vi "ScanPanel.vi"(8 "error in (no error)":errorcluster caption="entrée d'erreur (pas d'erreur)", 11 "BaseDevice.lvclass":refnum<class "BaseDevice.lvclass">) -> (0 "error out":errorcluster caption="sortie d'erreur", 3 "BaseDevice.lvclass Out":refnum<class "BaseDevice.lvclass">)   [LabVIEW 2019, in "BaseDevice.lvclass"]
uses:
  BaseDevice.lvclass
  ScanPos.ctl
panel:
  in  "AllerRetour":bool
  in  "UpdateScanTime":bool
  in  "MainProgQ":refnum<queue>
  in  "MainProgQEvent":refnum<user-event>
  in  "Reinit":bool caption="Reinit. à la fin"
  in  "Bidir":bool
  out "Positions":dbl[](array[numeric])
  in  "Modèle":u16(ring) caption="Modèle de Balayage"
  in  "CréerMod":bool
  in  "Debut":dbl caption="Début"
  in  "Fin":dbl
  in  "Increment":dbl=inf
  in  "ModRap":bool caption="Modèle Rapide"
  in  "Stop":bool
  out "Init Program":bool
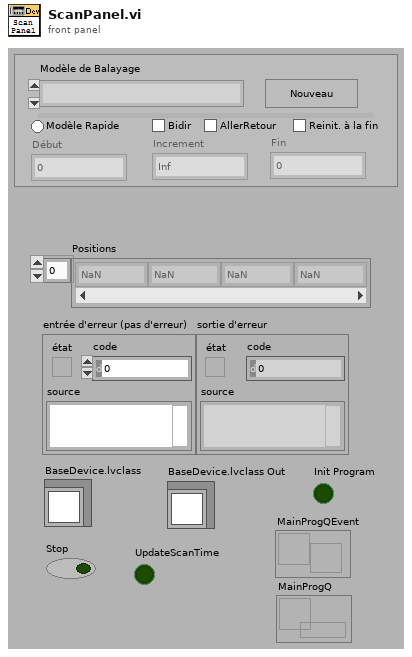
[diagram p1: front panel]
types:
  T1 = typedef "ScanPos.ctl" = cluster{"Debut":dbl, "Increment":dbl, "Fin":dbl, "Positions":dbl[], "Bidir":bool, "ModelRap":bool}
  T2 = enum16{"Enable", "Disable", "DisAndGrayed", "ReinitToDefVal"}
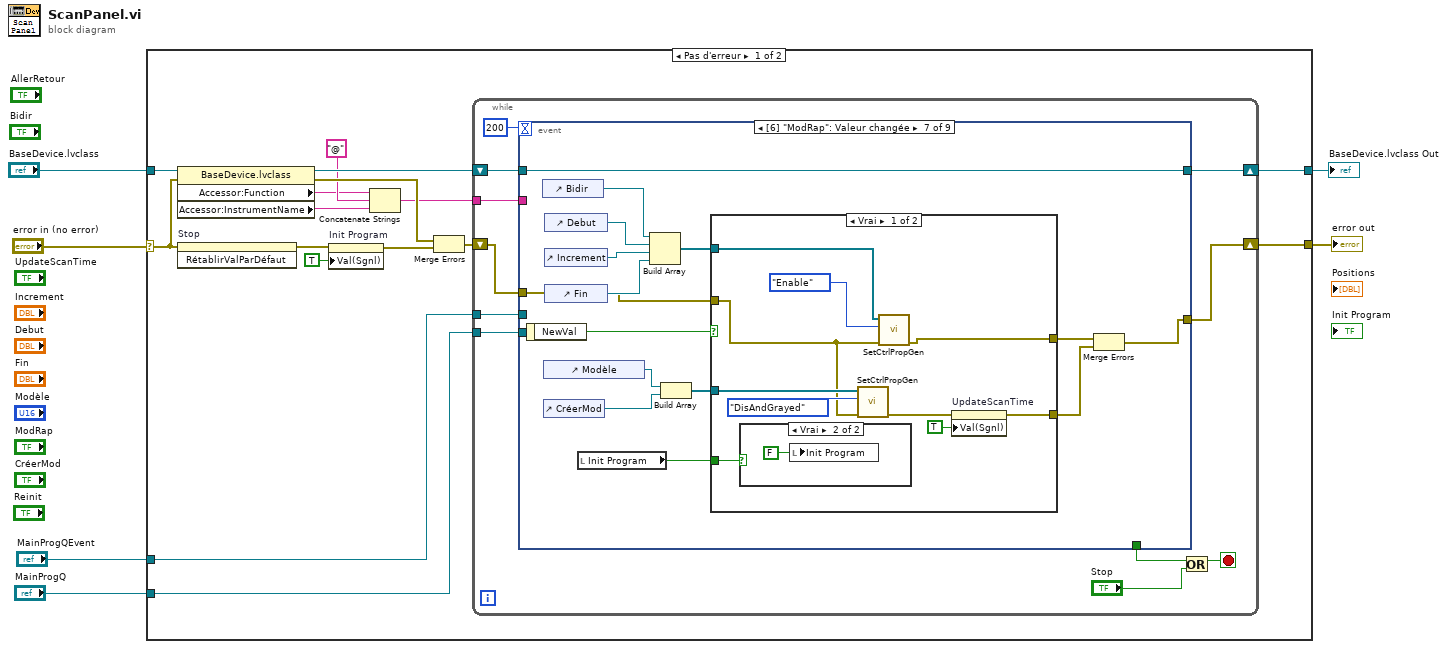
[diagram p0: block diagram]
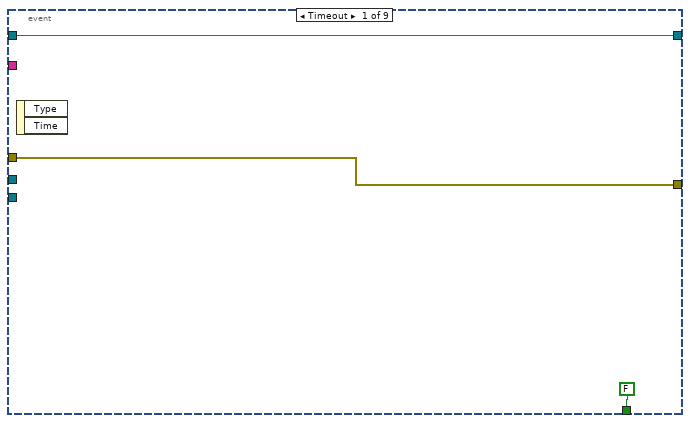
[diagram p2: hidden frame]
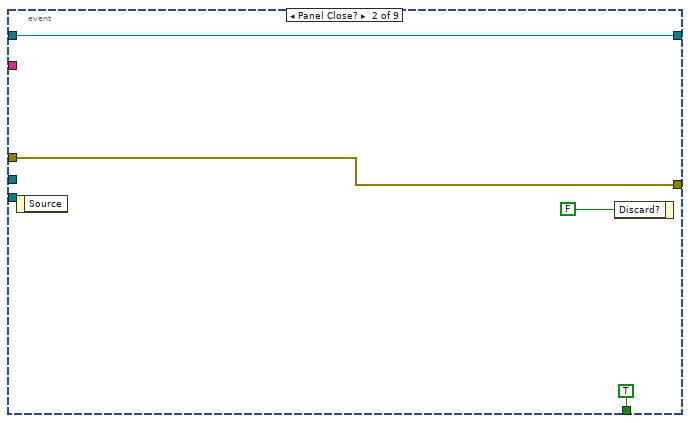
[diagram p3: hidden frame]
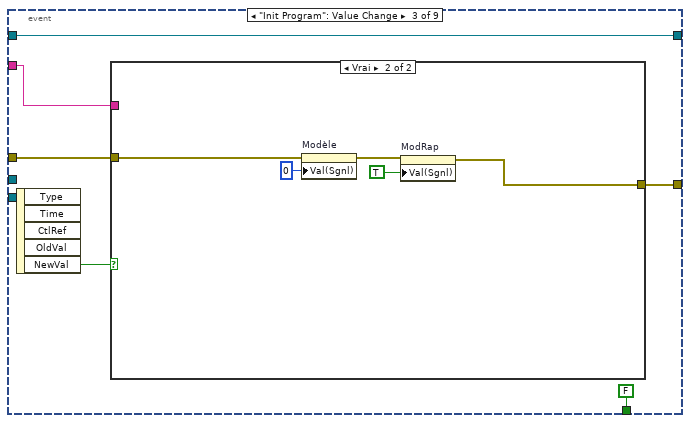
[diagram p4: hidden frame]
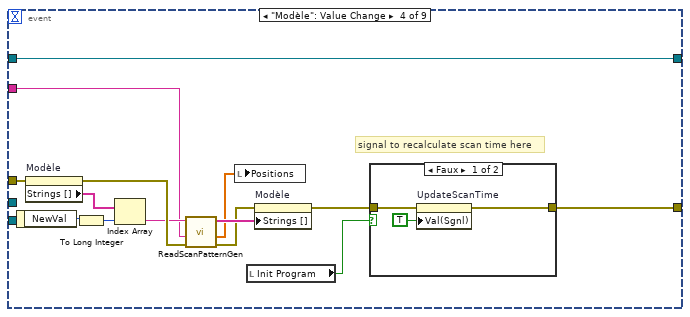
[diagram p6: hidden frame]
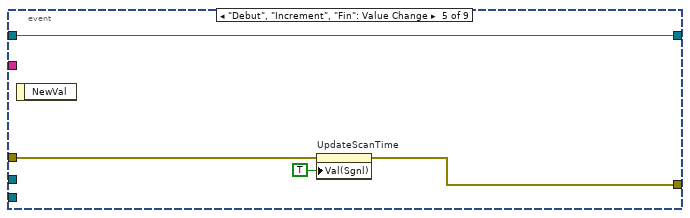
[diagram p8: hidden frame]
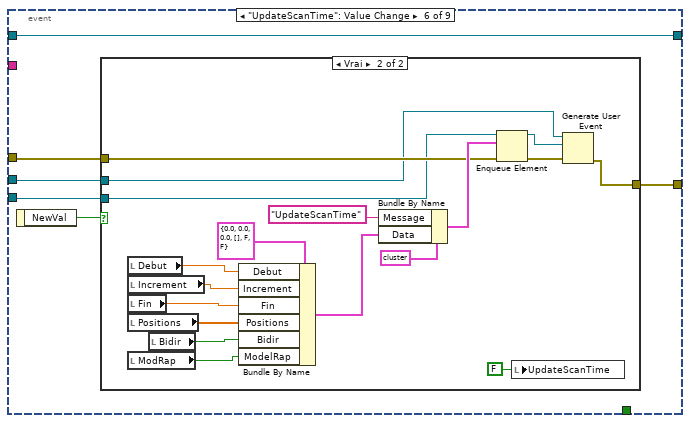
[diagram p9: hidden frame]
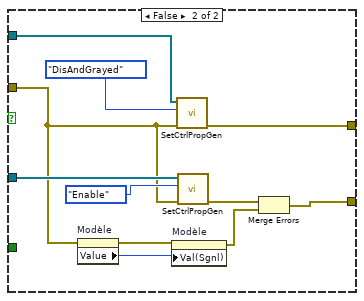
[diagram p12: hidden frame]
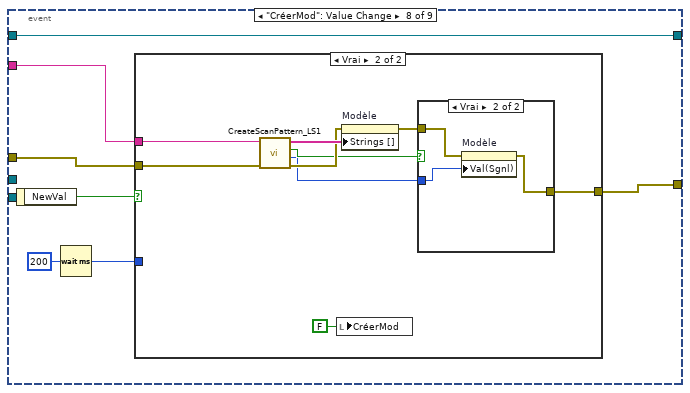
[diagram p13: hidden frame]
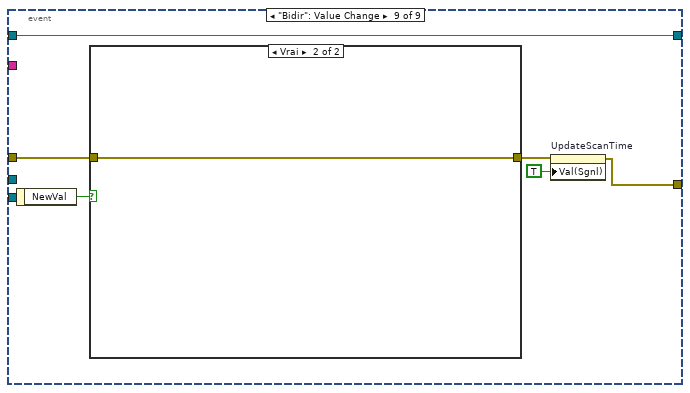
[diagram p16: hidden frame]
diagram:
  n1 = case shown="Pas d'erreur" "error in (no error)" {
    selector: "error in (no error)" -> [w16 w167]
    tunnel: [w22 w167] -> w5
    tunnel: "BaseDevice.lvclass" -> [w21 w166]
    tunnel: [w19 w166] -> w3
    tunnel: "MainProgQEvent" -> [w8 _]
    tunnel: "MainProgQ" -> [w7 _]
    frame No Error {
      n2 = property class="BaseDevice.lvclass"(reference=w21, error in=w16) -> (reference out=w17:refnum<class "BaseDevice.lvclass">, error out=w14:errorcluster, "Accessor:Function"=w11:string, "Accessor:InstrumentName"=w10:string)
      n3 = invoke on="Stop" class="Bool (strict)" method="RétablirValParDéfaut"(error in=w16) -> (error out=w18:errorcluster)  [unwired: 2 in, 2 out]
      n4 = property on="Init Program" class="Bool (strict)"(error in=w18, "Val(Sgnl)"=TRUE ("Valeur (Signalisation)")) -> (error out=w15:errorcluster)  [unwired: 1 in, 1 out]
      n5 = Concatenate Strings(w11, "@" ("chaîne"), w10) -> (w9:string)
      n6 = Merge Errors(w14, w15) -> (w13:errorcluster)
      n7 = while {
        shift-right: [w32] -> w22
        shift-left: w13 -> [w25]
        shift-right: [w29] -> w19
        shift-left: w17 -> [w31]
        tunnel: w9 -> [w26]
        tunnel: w8 -> [w24]
        tunnel: w7 -> [w23]
        stop <- w28 stop-if-true
        n8 = event shown="[6] \"ModRap\": Valeur changée" {
          selector: _ -> [_ _ _ _ _ _ _ _ _]
          dyn-events: _ -> [_ _ _ _ _ _ _ _ _]
          timeout: 200 -> [_ _ _ _ _ _ _ _ _]
          tunnel: w25 -> [w34 w38 w45 w66 w73 w80 w108 w138 w161]
          tunnel: [w34 w38 w44 w55 w72 w76 w102 w137 w159] -> w32
          tunnel: w31 -> [w35 w37 w43 w56 w74 w79 w107 w140 w162]
          tunnel: [FALSE TRUE FALSE _ _ _ _ _ _] -> w30
          tunnel: [w35 w37 w43 w56 w74 w79 w107 w140 w162] -> w29
          tunnel: w26 -> [_ _ w41 w57 _ _ _ w139 _]
          tunnel: w24 -> [_ _ _ _ _ w78 _ _ _]
          tunnel: w23 -> [_ _ _ _ _ w77 _ _ _]
          event Timeout {
            n9 = event-data() -> ()  [unwired: 1 in, 2 out]
          }
          event Panel Close? {
            n10 = event-data() -> ()  [unwired: 1 in, 1 out]
            n11 = event-data("Discard?"=FALSE ("Rejeter ?")) -> ()  [unwired: 1 in, 1 out]
          }
          event "Init Program": Value Change {
            n12 = event-data() -> ("NewVal"=w46:bool)  [unwired: 1 in, 4 out]
            n13 = case shown="Vrai" w46 {
              tunnel: w41 -> [_ _]
              tunnel: w45 -> [w47 w50]
              tunnel: [w47 w52] -> w44
              frame False {
              }
              frame True {
                n14 = property on="Modèle" class="MDér (strict)"(error in=w50, "Val(Sgnl)"=u16 0 ("Valeur (Signalisation)")) -> (error out=w49:errorcluster)  [unwired: 1 in, 1 out]
                n15 = property on="ModRap" class="Bool (strict)"(error in=w49, "Val(Sgnl)"=TRUE ("ModRap")) -> (error out=w52:errorcluster)  [unwired: 1 in, 1 out]
              }
            }
          }
          event "Modèle": Value Change {
            # "signal to recalculate scan time here"
            n16 = event-data() -> ("NewVal"=w64:u16)  [unwired: 1 in]
            n17 = property on="Modèle" class="MDér (strict)"(error in=w66) -> (error out=w62:errorcluster, "Strings []"=w63:string[])  [unwired: 1 in, 1 out]
            n18 = To Long Integer(number=w64) -> (32bit integer=w65:i32)
            n19 = Index Array(array=w63, index=w65) -> (element=w61:string)
            n20 = call <userlib>:"ReadScanPatternGen.vi"("Error in"=w62, "VarParam"=w57, "Modèle"=w61) -> ("Error out"=w59:errorcluster, "Positions"=w58:dbl[], "Modèles"=w60:string[])  [unwired: 2 in]
            n21 = local write "Positions"(w58) -> ()
            n22 = local read "Init Program"() -> (w53:bool)
            n23 = property on="Modèle" class="MDér (strict)"(error in=w59, "Strings []"=w60) -> (error out=w54:errorcluster)  [unwired: 1 in, 1 out]
            n24 = case shown="Faux" w53 {
              tunnel: [w69 w70] -> w55
              tunnel: w54 -> [w68 w70]
              frame False {
                n25 = property on="UpdateScanTime" class="Bool (strict)"(error in=w68, "Val(Sgnl)"=TRUE ("Value (Signaling)")) -> (error out=w69:errorcluster)  [unwired: 1 in, 1 out]
              }
              frame True {
              }
            }
          }
          event "Debut", "Increment", "Fin": Value Change {
            n26 = event-data() -> ()  [unwired: 1 in, 1 out]
            n27 = property on="UpdateScanTime" class="Bool (strict)"(error in=w73, "Val(Sgnl)"=TRUE ("Value (Signaling)")) -> (error out=w72:errorcluster)  [unwired: 1 in, 1 out]
          }
          event "UpdateScanTime": Value Change {
            n28 = event-data() -> ("NewVal"=w75:bool)  [unwired: 1 in]
            n29 = case shown="Vrai" w75 {
              tunnel: w80 -> [w81 w94]
              tunnel: w78 -> [_ w93]
              tunnel: w77 -> [_ w92]
              tunnel: [w81 w91] -> w76
              frame False {
              }
              frame True {
                n30 = local read "Debut"() -> (w84:dbl)
                n31 = local read "Increment"() -> (w90:dbl)
                n32 = local read "Fin"() -> (w89:dbl)
                n33 = local read "Positions"() -> (w88:dbl[])
                n34 = local read "ModRap"() -> (w83:bool)
                n35 = local read "Bidir"() -> (w85:bool)
                n36 = Bundle By Name(cluster=T1 {"Debut"=0.0, "Increment"=0.0, "Fin"=0.0, "Positions"=[], "Bidir"=FALSE, "ModelRap"=FALSE}, "Debut"=w84, "Increment"=w90, "Fin"=w89, "Positions"=w88, "Bidir"=w85, "ModelRap"=w83) -> (w86:T1)
                n37 = Bundle By Name(cluster=cluster{"Message":string, "Data":variant, i32} {"Message"="", "Data"=variant, 0} ("élément"), "Message"="UpdateScanTime", "Data"=w86) -> (w98:cluster{"Message":string, "Data":variant, i32})
                n38 = Enqueue Element(queue=w92, element=w98, error in (no error)=w94) -> (queue out=w97:refnum<queue>, error out=w96:errorcluster)  [unwired: 1 in, 1 out]
                n39 = local write "UpdateScanTime"(FALSE ("UpdateScanTime")) -> ()
                n40 = Generate User Event(user event=w93, event data cluster=w97, error in=w96) -> (error out=w91:errorcluster)  [unwired: 1 in, 1 out]
              }
            }
          }
          event "ModRap": Value Change {
            n41 = event-data() -> ("NewVal"=w106:bool)  [unwired: 1 in]
            n42 = control-ref of="Bidir"() -> (w101:refnum<vi>)
            n43 = control-ref of="Modèle"() -> (w110:refnum<vi>)
            n44 = control-ref of="CréerMod"() -> (w109:refnum<vi>)
            n45 = control-ref of="Debut"() -> (w114:refnum<vi>)
            n46 = control-ref of="Increment"() -> (w113:refnum<vi>)
            n47 = control-ref of="Fin"() -> (w112:refnum<vi>)
            n48 = local read "Init Program"() -> (w100:bool)
            n49 = Build Array(w101, w114, w113, w112) -> (w111:refnum<vi>[])
            n50 = Build Array(w110, w109) -> (w105:refnum<vi>[])
            n51 = case shown="Vrai" w106 {
              tunnel: w111 -> [w124 w136]
              tunnel: w108 -> [w120 w130]
              tunnel: w105 -> [w121 w133]
              tunnel: [w119 w132] -> w104
              tunnel: [w118 w126] -> w103
              tunnel: w100 -> [w116 _]
              frame True {
                n52 = case shown="Vrai" w116 {
                  frame False {
                  }
                  frame True {
                    n53 = local write "Init Program"(FALSE ("Value (Signaling)")) -> ()
                  }
                }
                n54 = call <userlib>:"SetCtrlPropGen.vi"("Error in"=w120, "Énum"=T2."DisAndGrayed", "Controls"=w121) -> ("Error out"=w115:errorcluster)  [unwired: 3 in, 1 out]
                n55 = call <userlib>:"SetCtrlPropGen.vi"("Error in"=w120, "Énum"=T2."Enable", "Controls"=w124) -> ("Error out"=w119:errorcluster)  [unwired: 3 in, 1 out]
                n56 = property on="UpdateScanTime" class="Bool (strict)"(error in=w115, "Val(Sgnl)"=TRUE ("Value (Signaling)")) -> (error out=w118:errorcluster)  [unwired: 1 in, 1 out]
              }
              frame False {
                n57 = property on="Modèle" class="MDér (strict)"(error in=w130) -> (error out=w129:errorcluster, "Value"=w131:u16)  [unwired: 1 in, 1 out]
                n58 = property on="Modèle" class="MDér (strict)"(error in=w129, "Val(Sgnl)"=w131) -> (error out=w127:errorcluster)  [unwired: 1 in, 1 out]
                n59 = call <userlib>:"SetCtrlPropGen.vi"("Error in"=w130, "Énum"=T2."DisAndGrayed", "Controls"=w136) -> ("Error out"=w132:errorcluster)  [unwired: 3 in, 1 out]
                n60 = call <userlib>:"SetCtrlPropGen.vi"("Error in"=w130, "Énum"=T2."Enable", "Controls"=w133) -> ("Error out"=w128:errorcluster)  [unwired: 3 in, 1 out]
                n61 = Merge Errors(w128, w127) -> (w126:errorcluster)
              }
            }
            n62 = Merge Errors(w104, w103) -> (w102:errorcluster)
          }
          event "CréerMod": Value Change {
            n63 = event-data() -> ("NewVal"=w143:bool)  [unwired: 1 in]
            n64 = Wait (ms)(milliseconds to wait=u32 200 ("attente (ms)")) -> (millisecond timer value=w142:u32)
            n65 = case shown="Vrai" w143 {
              tunnel: w142 -> [_ _]
              tunnel: w139 -> [_ w152]
              tunnel: w138 -> [w144 w151]
              tunnel: [w144 w147] -> w137
              frame False {
              }
              frame True {
                n66 = call "CreateScanPattern_LS1.vi"("Error in"=w151, "VarParam"=w152) -> ("Error out"=w149:errorcluster, "ModèleSauv"=w145:i32, "SavedOK"=w146:bool, "Modèles out"=w150:string[])  [unwired: 6 in]
                n67 = local write "CréerMod"(FALSE ("CréerMod")) -> ()
                n68 = property on="Modèle" class="MDér (strict)"(error in=w149, "Strings []"=w150) -> (error out=w148:errorcluster)  [unwired: 1 in, 1 out]
                n69 = case shown="Vrai" w146 {
                  tunnel: w148 -> [w154 w157]
                  tunnel: [w154 w156] -> w147
                  tunnel: w145 -> [_ w155]
                  frame False {
                  }
                  frame True {
                    n70 = property on="Modèle" class="MDér (strict)"(error in=w157, "Val(Sgnl)"=w155) -> (error out=w156:errorcluster)  [unwired: 1 in, 1 out]
                  }
                }
              }
            }
          }
          event "Bidir": Value Change {
            n71 = event-data() -> ("NewVal"=w163:bool)  [unwired: 1 in]
            n72 = case shown="Vrai" w163 {
              tunnel: [w164 w165] -> w160
              tunnel: w161 -> [w164 w165]
              frame False {
              }
              frame True {
              }
            }
            n73 = property on="UpdateScanTime" class="Bool (strict)"(error in=w160, "Val(Sgnl)"=TRUE ("Value (Signaling)")) -> (error out=w159:errorcluster)  [unwired: 1 in, 1 out]
          }
        }
        n74 = Or(x=w30, y="Stop") -> (x .or. y?=w28:bool)
      }
    }
    frame Error {
    }
  }
  "error out" <- w5
  "BaseDevice.lvclass Out" <- w3
